vi "Run All Unit Tests.vi"(7 "Main VI":path, 8 "Error In":errorcluster, 9 "Grader Result in":T6, 10 "Challenge Config":T5, 11 "VIChallenge Config":T1={"AWS Credentials"={"AWSAccessKeyId"="", "Secret Key"=""}, "AWS Account Number"="", "SQS Jobs"=refnum, "SQS Status"=refnum, "Source Dir"=path "", "Working Dir"=path "", "Output Dir"=path "", "Archive Dir"=path "", "job"={"job_id"="", "challenge_id"="", "user_id"="", "s3_source_bucket"="", "s3_source_directory"="", "s3_source_filename"="", "status_queue_name"="", "username"=""}, "Database Ref"=refnum, "Challenge Dir"=path "", "Challenges"=[]}) -> (0 "Error Out":errorcluster, 1 "Grader Result":T6, 2 "Challenge Config":T5, 3 "VIChallenge Config":T1)   [LabVIEW 2013, in "VIChallenge.lvlib"]
doc: "This VI runs all unit tests for the given challenge and returns a single result."
uses:
  <vilib>/LabVIEW Hacker/VIChallenge/VIChallenge.lvlib
  <vilib>/LabVIEW Hacker/VIChallenge/Private/Grader/Type Defs/Grader Result.ctl
  <vilib>/LabVIEW Hacker/VIChallenge/Private/Type Defs/Database/Score.ctl
  <vilib>/LabVIEW Hacker/VIChallenge/Private/Grader/Type Defs/UTF Status.ctl
  <vilib>/LabVIEW Hacker/VIChallenge/Private/Grader/Type Defs/Challenge.ctl
  <vilib>/LabVIEW Hacker/VIChallenge/Private/Type Defs/VIChallenge Config.ctl
  <vilib>/National Instruments/NI Amazon Web Services (AWS) Toolkit for LabVIEW/SQS/VI Source/AWS SQS Class/AWS_SQS.lvclass
  <vilib>/National Instruments/NI Amazon Web Services (AWS) Toolkit for LabVIEW/AWS Core Lib/VI Source/Canonicals/AWS_Core Canonical Credentials/Canonical Credentials.lvclass
  <vilib>/National Instruments/NI Amazon Web Services (AWS) Toolkit for LabVIEW/AWS Core Lib/VI Source/Canonicals/AWS_Core Canonical Required Parameters/Canonical Required Parameters.lvclass
  <vilib>/National Instruments/NI Amazon Web Services (AWS) Toolkit for LabVIEW/SQS/VI Source/Canonicals/Canonical CreateQueue/Canonical CreateQueue.lvclass
  <vilib>/National Instruments/NI Amazon Web Services (AWS) Toolkit for LabVIEW/SQS/VI Source/Canonicals/Canonical ListQueues/Canonical ListQueues.lvclass
  <vilib>/National Instruments/NI Amazon Web Services (AWS) Toolkit for LabVIEW/SQS/VI Source/Canonicals/Canonical AddPermission/Canonical AddPermission.lvclass
  <vilib>/National Instruments/NI Amazon Web Services (AWS) Toolkit for LabVIEW/SQS/VI Source/Canonicals/Canonical ChangeMessageVisibility/Canonical ChangeMessageVisibility.lvclass
  <vilib>/National Instruments/NI Amazon Web Services (AWS) Toolkit for LabVIEW/SQS/VI Source/Canonicals/Canonical ChangeMessageVisibilityBatch/Canonical ChangeMessageVisibilityBatch.lvclass
  <vilib>/National Instruments/NI Amazon Web Services (AWS) Toolkit for LabVIEW/SQS/VI Source/Canonicals/Canonical DeleteMessage/Canonical DeleteMessage.lvclass
  <vilib>/National Instruments/NI Amazon Web Services (AWS) Toolkit for LabVIEW/SQS/VI Source/Canonicals/Canonical DeleteMessageBatch/Canonical DeleteMessageBatch.lvclass
  <vilib>/National Instruments/NI Amazon Web Services (AWS) Toolkit for LabVIEW/SQS/VI Source/Canonicals/Canonical GetQueueAttributes/Canonical GetQueueAttributes.lvclass
  <vilib>/National Instruments/NI Amazon Web Services (AWS) Toolkit for LabVIEW/SQS/VI Source/Canonicals/Canonical GetQueueUrl/Canonical GetQueueUrl.lvclass
  <vilib>/National Instruments/NI Amazon Web Services (AWS) Toolkit for LabVIEW/SQS/VI Source/Canonicals/Canonical ReceiveMessage/Canonical ReceiveMessage.lvclass
  <vilib>/National Instruments/NI Amazon Web Services (AWS) Toolkit for LabVIEW/SQS/VI Source/Canonicals/Canonical RemovePermission/Canonical RemovePermission.lvclass
  <vilib>/National Instruments/NI Amazon Web Services (AWS) Toolkit for LabVIEW/SQS/VI Source/Canonicals/Canonical SendMessage/Canonical SendMessage.lvclass
  <vilib>/National Instruments/NI Amazon Web Services (AWS) Toolkit for LabVIEW/SQS/VI Source/Canonicals/Canonical SendMessageBatch/Canonical SendMessageBatch.lvclass
  <vilib>/National Instruments/NI Amazon Web Services (AWS) Toolkit for LabVIEW/SQS/VI Source/Canonicals/Canonical SetQueueAttributes/Canonical SetQueueAttributes.lvclass
  <vilib>/National Instruments/NI Amazon Web Services (AWS) Toolkit for LabVIEW/AWS Core Lib/VI Source/Typedefs/AWS_AWS Credentials.ctl
  <vilib>/LabVIEW Hacker/VIChallenge/Private/Type Defs/JSON_job.ctl
  <vilib>/addons/database/Connection.llb/Conn ObjectReference.ctl
  <vilib>/utf/NI_UnitTestFramework.lvlib
  <vilib>/National Instruments/NI Amazon Web Services (AWS) Toolkit for LabVIEW/AWS Core Lib/VI Source/AWS_Core.lvlib
  <vilib>/addons/database/NI_Database_API.lvlib
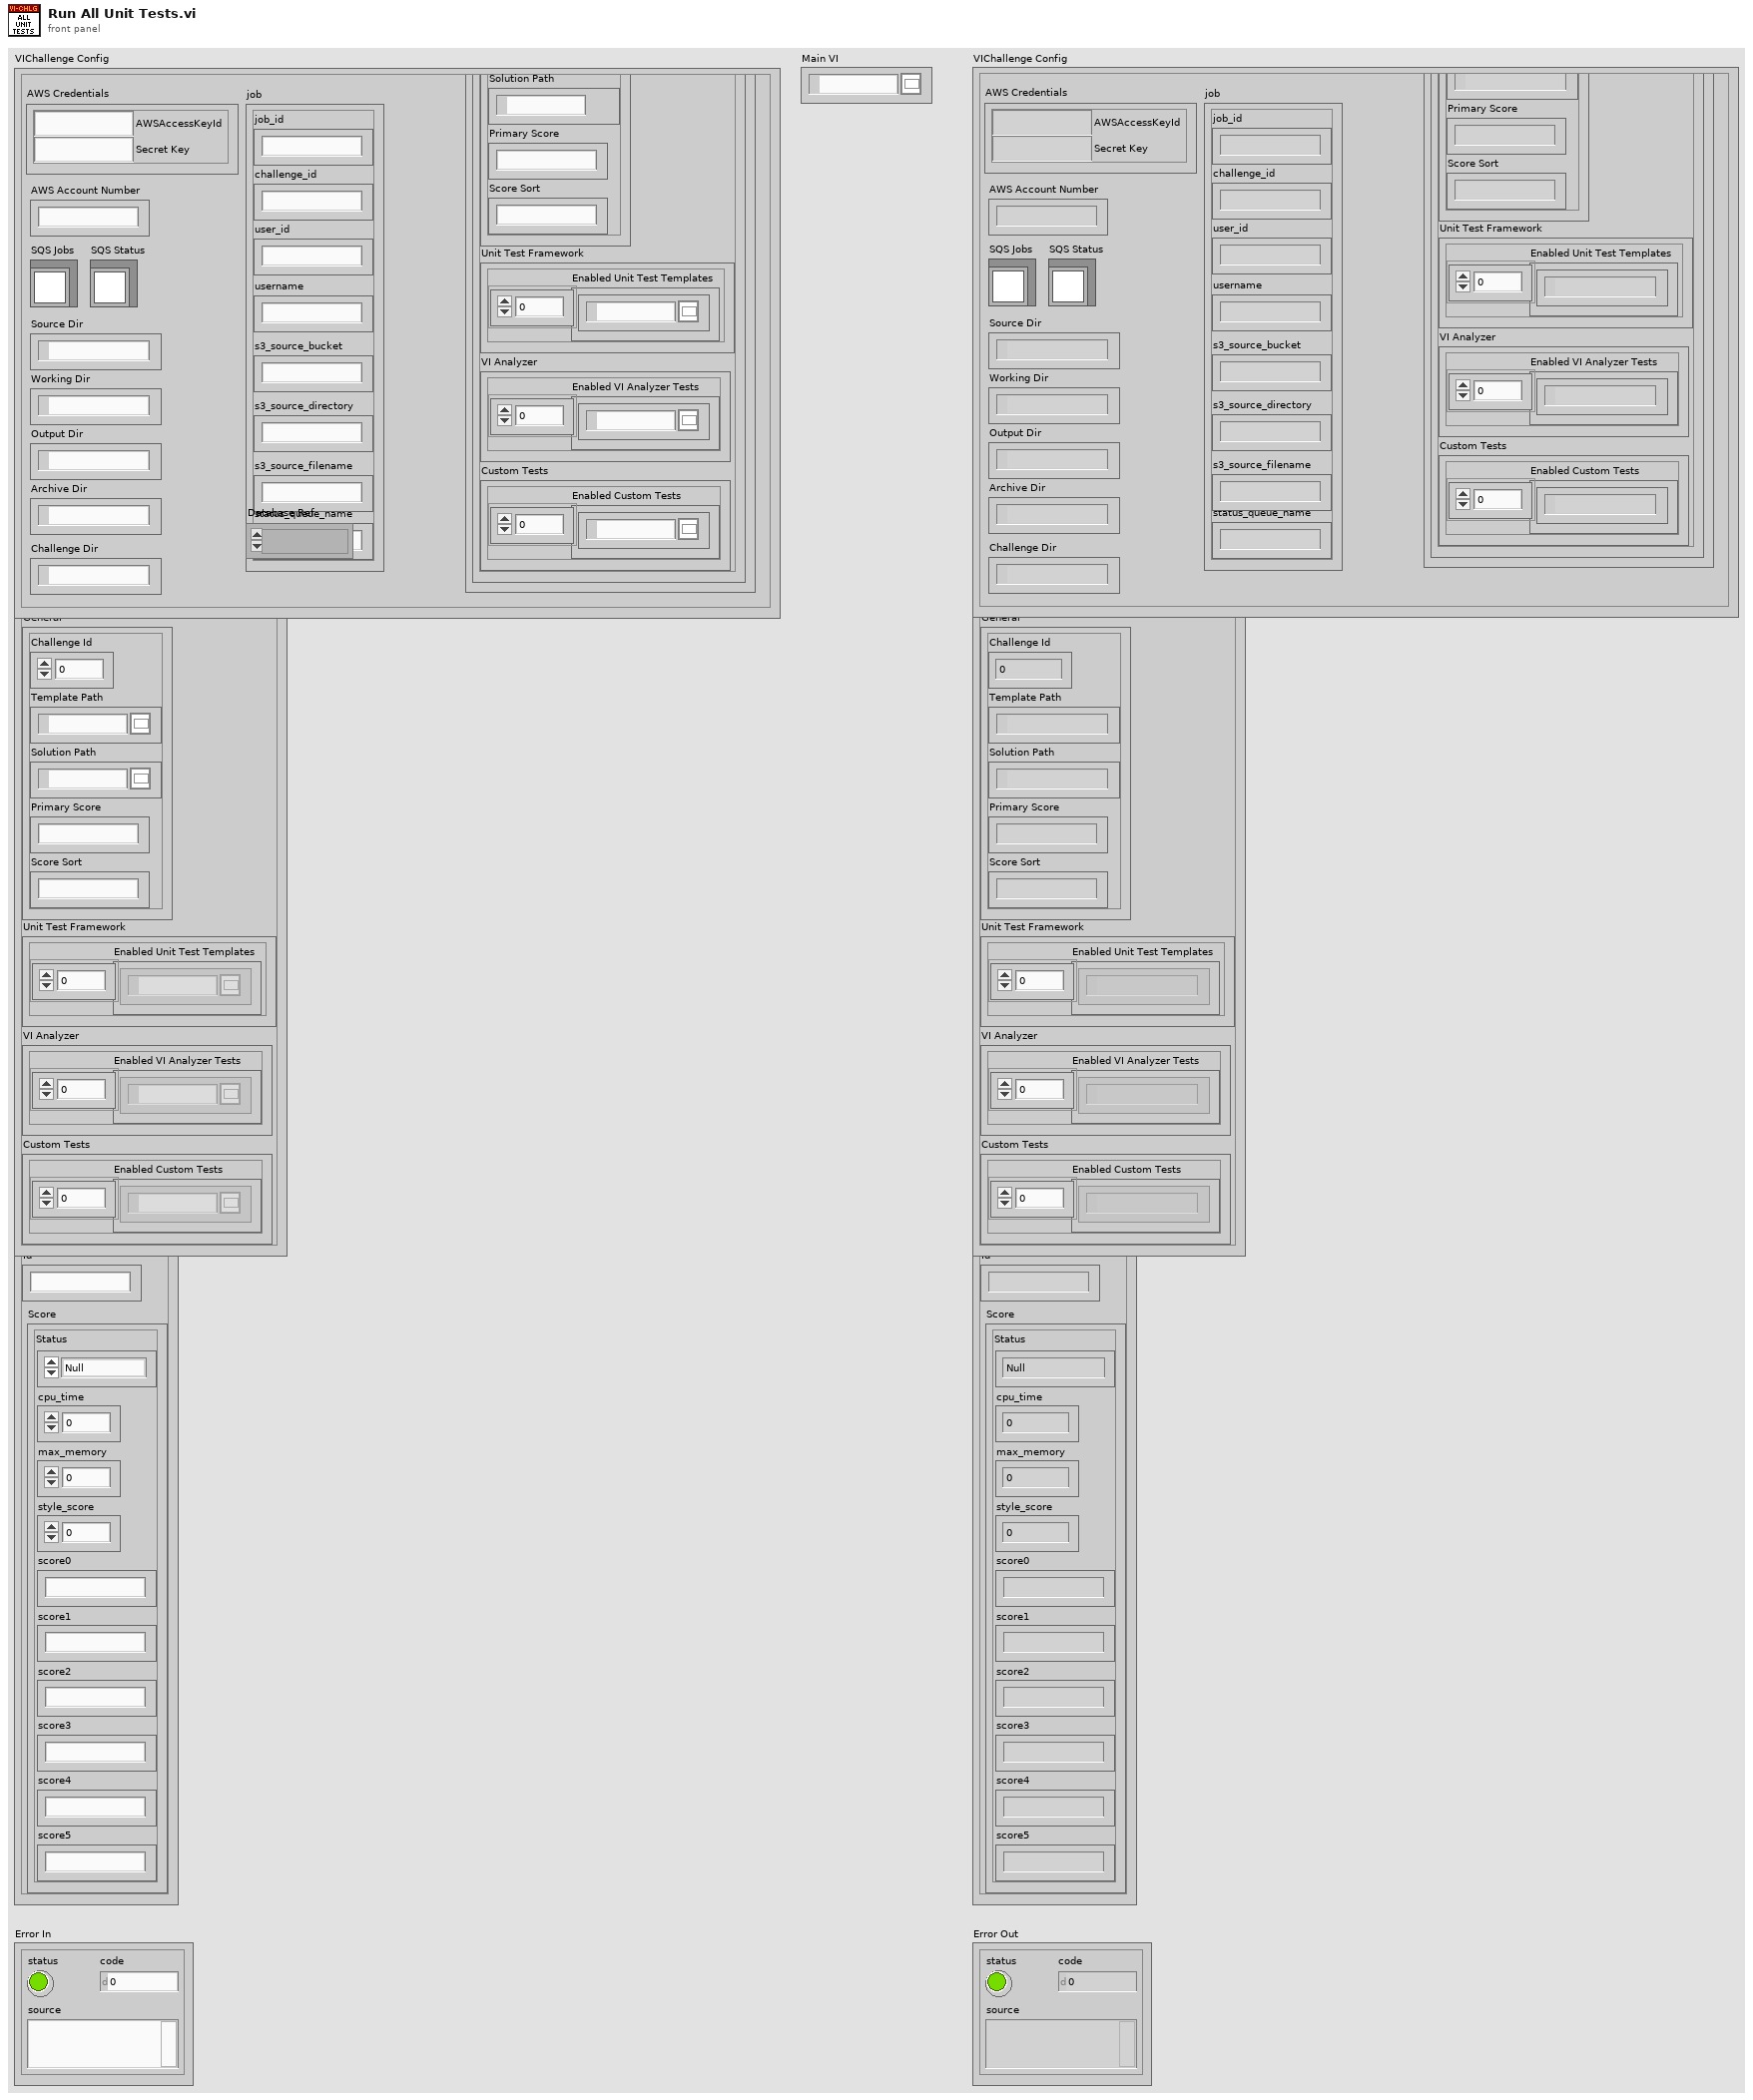
[diagram p1: front panel]
types:
  T1 = typedef "VIChallenge.lvlib/VIChallenge Config.ctl" = cluster{"AWS Credentials":T2, "AWS Account Number":string, "SQS Jobs":refnum<class "AWS_SQS.lvclass">, "SQS Status":refnum<class "AWS_SQS.lvclass">, "Source Dir":path, "Working Dir":path, "Output Dir":path, "Archive Dir":path, "job":T3, "Database Ref":T4, "Challenge Dir":path, "Challenges":T5[]}
  T2 = typedef "AWS_Core.lvlib/AWS_AWS Credentials.ctl" = cluster{"AWSAccessKeyId":string, "Secret Key":string}
  T3 = typedef "VIChallenge.lvlib/JSON_job.ctl" = cluster{"job_id":string, "challenge_id":string, "user_id":string, "s3_source_bucket":string, "s3_source_directory":string, "s3_source_filename":string, "status_queue_name":string, "username":string}
  T4 = typedef "NI_Database_API.lvlib/Conn ObjectReference.ctl" = refnum<k1>
  T5 = typedef "VIChallenge.lvlib/Challenge.ctl" = cluster{"General":cluster{"Challenge Id":i32, "Template Path":path, "Solution Path":path, "Primary Score":string, "Score Sort":string}, "Unit Test Framework":cluster{"Enabled Unit Test Templates":path[]}, "VI Analyzer":cluster{"Enabled VI Analyzer Tests":path[]}, "Custom Tests":cluster{"Enabled Custom Tests":path[]}}
  T6 = typedef "VIChallenge.lvlib/Grader Result.ctl" = cluster{"Id":string, "Score":T7}
  T7 = typedef "VIChallenge.lvlib/Score.ctl" = cluster{"Status":T8, "cpu_time":i32, "max_memory":i32, "style_score":i32, "score0":string, "score1":string, "score2":string, "score3":string, "score4":string, "score5":string}
  T8 = typedef "VIChallenge.lvlib/UTF Status.ctl" = enum16{"Null", "Passed", "Failed", "Error", "Skipped", "Not Processed"}
  T9 = typedef "NI_UnitTestFramework.lvlib/utf_test_result_overall.ctl" = cluster{"utf results out":T10[], "untested VIs":cluster{"VI path":path, "code coverage":T19, "vi hierarchy":string[]}[], "project file path":path, "system information":string}
  T10 = typedef "NI_UnitTestFramework.lvlib/utf_test_result_testfile.ctl" = cluster{"test case":T11[], "test status":T12, "test path":path, "setup VI":path, "teardown VI":path, "code coverage":T19, "start time":timestamp, "end time":timestamp, "test hierarchy":string[], "VI path":path, "VI timestamp":timestamp, "VI rev hist":i32, "requirements ID":string, "array brackets":string, "name separator":string, "errors":T20[], "paragraph header":string, "result comment":string, "vi hierarchy":string[], "subVI coverage info":T19[], "subVI info":T22[], "big array threshold":u32, "VI Index":i32, "Comment":string, "Dynamic Dispatch":bool, "User-defined test VI":path, "user-defined VI code coverage":T19}
  T11 = typedef "NI_UnitTestFramework.lvlib/utf_test_result_testcase.ctl" = cluster{"test result":T12, "run Times":T13[], "test case name":string, "requirements":string, "code coverage":T19, "subVI coverage info":T19[]}
  T12 = typedef "NI_UnitTestFramework.lvlib/utf_test_result.ctl" = enum16{"Passed", "Failed", "Error", "Skipped", "Not Processed"}
  T13 = typedef "NI_UnitTestFramework.lvlib/utf_test_result_troll_new.ctl" = cluster{"result (test)":T12, "Vector Result":T14[]}
  T14 = typedef "NI_UnitTestFramework.lvlib/utf_vector_result.ctl" = cluster{"time elapsed [ms]":u32, "result (test)":T12, "result (parameters)":T15[], "Used Vector Values":cluster{"Vector Name":string, "element":i32}[], "Executed Class Path":path, "Input":T18[]}
  T15 = typedef "NI_UnitTestFramework.lvlib/utf_test_result_failure.ctl" = cluster{"result":T12, "error message":string, "parameter name":string, "parameter value":variant, "parameters":variant[], "comparison":T16, "requirement ID":string, "VI":T17, "Used Vector Name":string}
  T16 = typedef "NI_UnitTestFramework.lvlib/utf_test_comparison_operators.ctl" = enum16{"=", "!=", ">", ">=", "<", "<=", "range", "symmetric tolerance", "asymmetric tolerance", "string contains", "string not contain", "array size", "string length", "array range", "by element", "array range (limit array)", "user-defined", "array contains", "array not contain", "vector length", "= (elm)", "!= (elm)", "= (case insensitive)", "!= (case insensitive)"}
  T17 = typedef "NI_UnitTestFramework.lvlib/utf_vi_tag.ctl" = enum16{"Setup VI", "VI under Test", "Teardown VI"}
  T18 = typedef "NI_UnitTestFramework.lvlib/utf_test_result_input_data.ctl" = cluster{"Name":string, "Input Value":variant[], "VI":T17, "Used Vector Index":i32}
  T19 = typedef "NI_UnitTestFramework.lvlib/utf_code_coverage.ctl" = cluster{"coverage":dbl, "diagram run flag":bool[]}
  T20 = typedef "NI_UnitTestFramework.lvlib/utf_error_data.ctl" = cluster{"error type":T21, "description":string}
  T21 = typedef "NI_UnitTestFramework.lvlib/utf_error_type.ctl" = enum16{"TestFileError", "VIError", "SetupVIError", "TearDownVIError", "OtherError"}
  T22 = typedef "NI_UnitTestFramework.lvlib/utf_subvi_info.ctl" = cluster{"Path":path, "Dependence VI":bool}
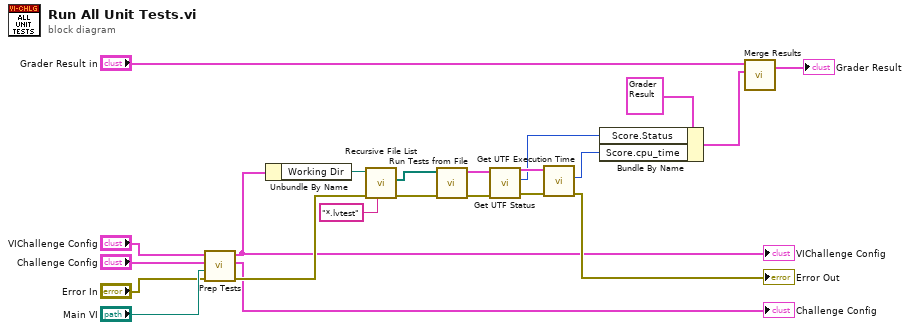
[diagram p0: block diagram]
diagram:
  n1 = call <vilib>:"Prep Tests.vi"("Error In"="Error In", "User Main VI"="Main VI", "Challenge Config"="Challenge Config", "VIChallenge Config"="VIChallenge Config") -> ("Error Out"=w22:errorcluster, "Challenge Config"=→"Challenge Config":T5, "VIChallenge Config"=w2:T1)  [unwired: 5 in]
  "VIChallenge Config" <- w2
  n2 = Unbundle By Name(w2) -> ("Working Dir"=w20:path)
  n3 = call <vilib>:"Recursive File List.vi"("pattern"="*.lvtest", "error in (no error)"=w22, "Folder Path"=w20) -> ("error out"=w21:errorcluster, "All Files in Dir"=w18:path[])  [unwired: 4 in, 3 out]
  n4 = call <vilib>:"Run Tests from File.vi"("error in (no error)"=w21, "test file paths"=w18) -> ("error out"=w17:errorcluster, "test results out"=w16:T9)  [unwired: 8 in]
  n5 = call <vilib>:"Get UTF Status.vi"("Error In"=w17, "UTF Results"=w16) -> ("Error Out"=w14:errorcluster, "Status"=w12:T8, "UTF Results"=w15:T9)  [unwired: 7 in]
  n6 = call <vilib>:"Get UTF Execution Time.vi"("Error In"=w14, "UTF Results"=w15) -> ("Error Out"=→"Error Out":errorcluster, "Execution Time (us)"=w13:i32)  [unwired: 7 in, 1 out]
  n7 = Bundle By Name(cluster=T6 {"Id"="", "Score"={"Status"=enum."Passed", "cpu_time"=-1, "max_memory"=-1, "style_score"=-1, "score0"="", "score1"="", "score2"="", "score3"="", "score4"="", "score5"=""}} ("Result 2"), "Score.Status"=w12, "Score.cpu_time"=w13) -> (w4:T6)
  n8 = call <vilib>:"Merge Results.vi"("Result 2"=w4, "Results 1"="Grader Result in") -> ("Results"=→"Grader Result":T6)  [unwired: 3 in]
